vi "Maxi Gauge-Convert Error1.vi"(3 "Errorwort1":u16) -> (0 "Error Text":string[](array[string]))   [LabVIEW 2012, in "Maxi Gauge.lvlib"]
uses:
  Maxi Gauge.lvlib
panel:
  in  "Error Tabel":string[][](table)=[["0", "WDT Watchdog Error"], ["1", "TSFK Task-Fail Error"], ["2", "IDLE IDCX System Error"], ["3", "STAC Stack Overflow Error"], ["4", "EPR Eprom-Error"], ["5", "RAM Ram Error"], ["6", "EEP EEprom Error"], ["7", "KEY Key Error"], ["8", "DISP Display Error"], ["9", ""], ["10", ""], ["11", ""], ["12", "STX Syntax Error"], ["13", "PAR invalid Parameter"], ["14", "HDW Hardware Error"], ["15", "FAT Fatal Error"]]
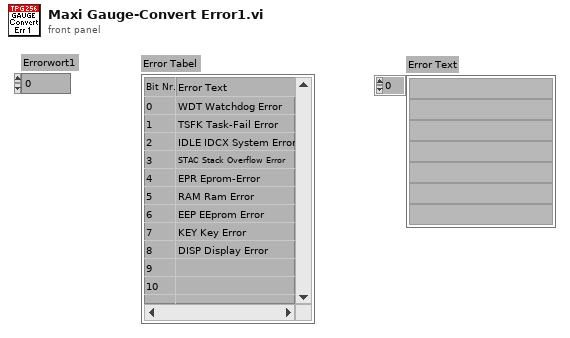
[diagram p1: front panel]
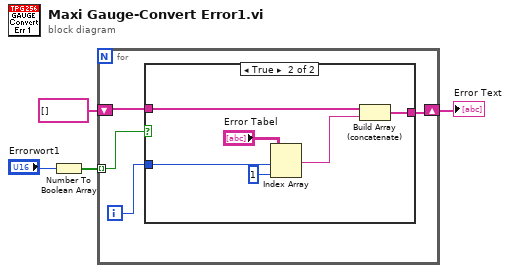
[diagram p0: block diagram]
diagram:
  n1 = Number To Boolean Array(number="Errorwort1") -> (Boolean array=w4:bool[])
  n2 = for {
    tunnel: w4 -> [w8] mode=indexing
    shift-right: [w5] -> w2
    shift-left: string[] [] -> [w6]
    i -> [w7]
    n3 = case shown="True" w8 {
      tunnel: w7 -> [_ w10]
      tunnel: w6 -> [w9 w13]
      tunnel: [w9 w11] -> w5
      frame False {
      }
      frame True {
        n4 = Index Array(array="Error Tabel", index (row)=w10, index (col)=1) -> (element=w12:string)
        n5 = Build Array (concatenate)(w13, w12) -> (w11:string[])
      }
    }
  }
  "Error Text" <- w2
